vi "Update Dynamic Shunt Default Values.vi"(8 "error in (no error)":errorcluster, 9 "Dynamic shunt?":bool, 10 "9237 in":refnum<class "9237.lvclass">, 11 "Node Ptr in":T1 format="%.0x") -> (0 "error out":errorcluster, 2 "9237 out":refnum<class "9237.lvclass">, 3 "Node Ptr out":T1 format="%.0x")   [LabVIEW 2019, in "Modules.lvlib" / "9237.lvclass"]
uses:
  9237.lvclass
  <vilib>/NI VeriStand/Custom Device API/Custom Device Item Ref.ctl
  9237.lvclass/9237.ctl
  RSI Module/Channel GUIDs.vi
  <vilib>/NI VeriStand/Custom Device Tools/Custom Device Utility Library/NI VeriStand - Search for Item by GUID.vi
  <vilib>/NI VeriStand/Custom Device Tools/Custom Device Utility Library/Custom Device Utility Library.lvlib
  RSI Module/RSI Module.lvclass
  <vilib>/NI VeriStand/Custom Device API/Custom Device API.lvlib
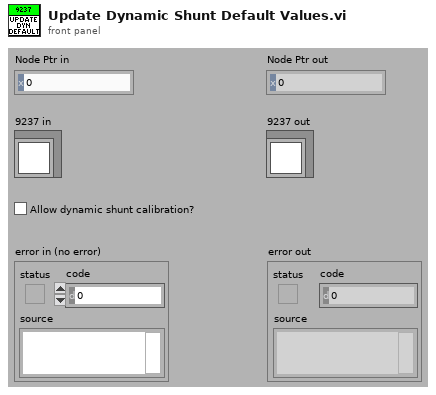
[diagram p1: front panel]
types:
  T1 = typedef "Custom Device API.lvlib/Custom Device Item Ref.ctl" = u64
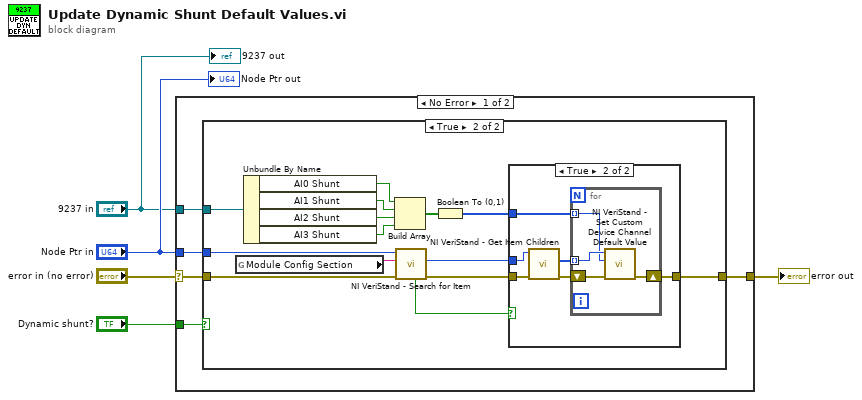
[diagram p0: block diagram]
diagram:
  n1 = case shown="No Error" "error in (no error)" {
    selector: "error in (no error)" -> [w7 w37]
    tunnel: [w6 w37] -> w4
    tunnel: "9237 in" -> [w9 _]
    tunnel: "Dynamic shunt?" -> [w10 _]
    tunnel: "Node Ptr in" -> [w8 _]
    frame No Error {
      n2 = case shown="True" w10 {
        tunnel: w9 -> [_ w13]
        tunnel: w8 -> [_ w21]
        tunnel: w7 -> [w11 w20]
        tunnel: [w11 w12] -> w6
        frame False {
        }
        frame True {
          n3 = global read "Channel GUIDs.vi" "Module Config Section"() -> (w25:string)
          n4 = Unbundle By Name(w13) -> ("AI0 Shunt"=w18:bool, "AI1 Shunt"=w17:bool, "AI2 Shunt"=w16:bool, "AI3 Shunt"=w15:bool)
          n5 = Build Array(w18, w17, w16, w15) -> (w19:bool[])
          n6 = call-poly <vilib>:"NI VeriStand - Search for Item.vi"("error in"=w20, "Item GUID"=w25, "Section Ref in"=w21) -> ("error out"=w23:errorcluster, "Item Ref"=w22:T1, "Found"=w24:bool)  [unwired: 5 in, 1 out]
          n7 = Boolean To (0,1)(Boolean=w19) -> (0, 1=w14:i16[])
          n8 = case shown="True" w24 {
            tunnel: w23 -> [w26 w32]
            tunnel: w22 -> [_ w31]
            tunnel: [w26 w29] -> w12
            tunnel: w14 -> [_ w27]
            frame False {
            }
            frame True {
              n9 = call <vilib>:"NI VeriStand - Get Item Children.vi"("error in (no error)"=w32, "Item Ref in"=w31) -> ("error out"=w30:errorcluster, "Child Refs"=w28:T1[])  [unwired: 6 in, 2 out]
              n10 = for {
                shift-right: [w35] -> w29
                shift-left: w30 -> [w36]
                tunnel: w28 -> [w34] mode=indexing
                tunnel: w27 -> [w33] mode=indexing
                n11 = call <vilib>:"NI VeriStand - Set Custom Device Channel Default Value.vi"("error in (no error)"=w36, "Default Value"=w33, "Channel Ref in"=w34) -> ("error out"=w35:errorcluster)  [unwired: 7 in, 1 out]
              }
            }
          }
        }
      }
    }
    frame Error {
    }
  }
  "error out" <- w4
  "9237 out" <- "9237 in"
  "Node Ptr out" <- "Node Ptr in"
